vi "Image to Printer.vi"(8 "error in (no error)":errorcluster, 11 "Control Ref Queue":T1) -> (0 "error out":errorcluster)   [LabVIEW 2017, in "3D Plot.lvclass"]
uses:
  <vilib>/Math Plots/3D Math Plots/3D Plot/3D Plot/3D Plot.lvclass
  <vilib>/Math Plots/3D Math Plots/3D Plot/Action String/3DMathPlot Ctrl Act Queue.ctl
  <vilib>/Math Plots/3D Math Plots/3D Plot/Action String/3DMathPlot Ctrl Act Cluster.ctl
  <vilib>/Math Plots/3D Math Plots/3D Plot/Action String/3DMathPlot State Class.ctl
  <vilib>/Math Plots/Plot Private Lib/NI_Math Plot Private Lib.lvlib
panel:
  in  "Print Image":picture
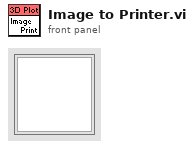
[diagram p1: front panel]
types:
  T1 = typedef "3DMathPlot Ctrl Act Queue.ctl" = refnum<queue>
  T2 = typedef "3DMathPlot Ctrl Act Cluster.ctl" = cluster{"3D Picture Control":refnum<vi>, "Render Window Refnum":refnum<vi>, "XY Graph":refnum<vi>, "Intensity Graph":refnum<vi>, "Color Legend Palette":refnum<vi>, "Projection Palette":refnum<vi>, "XControl  Ref":refnum<vi>, "Facade Ref":refnum<vi>, "Export Image Ref":refnum<vi>, "Clear Data Flag":bool, "Display State Change Class":T3}
  T3 = typedef "3DMathPlot State Class.ctl" = enum16{"Update All Objects (Undo)", "Update Light Object Only", "Update Axis Object Only", "Update Plot Object Only", "Update Cursor Object Only", "Update Axis Plot Cursor Objects", "No Update"}
  T4 = typedef "imagedata.ctl" = cluster{"image type":i32, "image depth":i32, "image":u8[], "mask":u8[], "colors":u32[], "Rectangle":cluster{"left":i16, "top":i16, "right":i16, "bottom":i16}}
  T5 = typedef "LVRectTypeDef.ctl" = cluster{"Left":i16, "Top":i16, "Right":i16, "Bottom":i16}
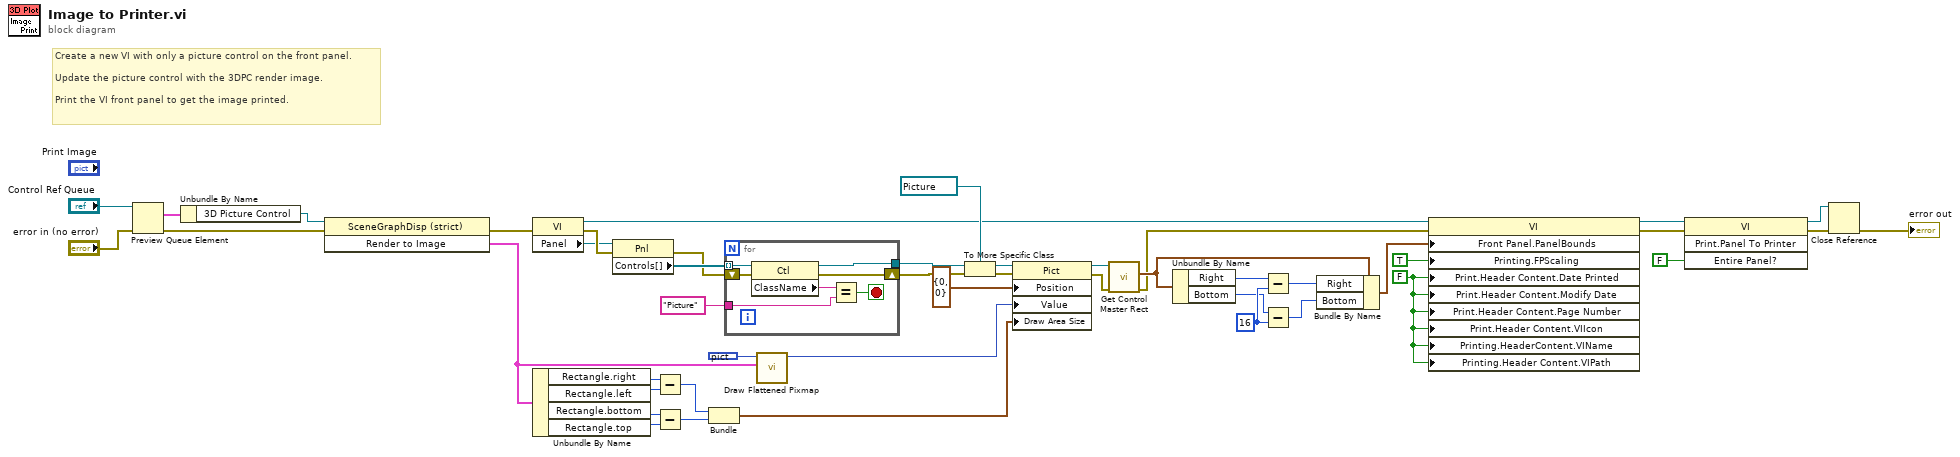
[diagram p0: block diagram]
diagram:
  w20 = i16 16
  w31 = FALSE ("Printing:Front Panel Scaling?")
  # "Create a new VI with only a picture control on the front panel.\n\nUpdate the picture control with the 3DPC render image.\n\nPrint the VI front panel to get the image printed."
  n1 = Preview Queue Element(queue="Control Ref Queue", error in (no error)="error in (no error)") -> (element=w28:T2, error out=w26:errorcluster)  [unwired: 3 out]
  n2 = Unbundle By Name(w28) -> ("3D Picture Control"=w27:refnum<vi>)
  n3 = invoke on="Invoke Node" class="SceneGraphDisp (strict)" method="Render to Image"(reference=w27, error in=w26) -> (error out=w13:errorcluster, "Get Image"=w29:T4)  [unwired: 1 in, 1 out]
  n4 = property class="VI"(error in=w13) -> (reference out=w14:refnum<vi>, error out=w16:errorcluster, "Panel"=w15:refnum<vi>)  [unwired: 1 in]
  n5 = Unbundle By Name(w29) -> ("Rectangle.right"=w38:i16, "Rectangle.left"=w40:i16, "Rectangle.bottom"=w37:i16, "Rectangle.top"=w39:i16)
  n6 = property class="Pnl"(reference=w15, error in=w16) -> (error out=w4:errorcluster, "Controls[]"=w6:refnum<vi>[])  [unwired: 1 out]
  n7 = Subtract(x=w38, y=w40) -> (x-y=w42:i16)
  n8 = Subtract(x=w37, y=w39) -> (x-y=w41:i16)
  n9 = Bundle(w42, w41) -> (w2:cluster{i16, i16})  [unwired: 1 out]
  n10 = for {
    tunnel: w6 -> [w53] mode=indexing
    tunnel: [w50] -> w5
    shift-right: [w48] -> w3
    shift-left: w4 -> [w49]
    tunnel: "Picture" -> [w47]
    stop <- w51 stop-if-true
    n11 = property class="Ctl"(reference=w53, error in=w49) -> (reference out=w50:refnum<vi>, error out=w48:errorcluster, "ClassName"=w52:string)
    n12 = Equal?(x=w52, y=w47) -> (x = y?=w51:bool)
  }
  n13 = call <vilib>:"Draw Flattened Pixmap.vi"("image data"=w29, "picture"=picture data[5B]) -> ("new picture"=w8:picture)  [unwired: 7 out]
  n14 = To More Specific Class(target class=refnum<vi> refnum ("reference"), reference=w5, error in=w3) -> (specific class reference=w24:refnum<vi>, error out=w25:errorcluster)
  n15 = property class="Pict"(reference=w24, error in=w25, "Position"=cluster{"Horizontal":i16, "Vertical":i16} {"Horizontal"=0, "Vertical"=0} ("relative position/next to refnum"), "Value"=w8, "Draw Area Size"=w2) -> (reference out=w12:refnum<vi>, error out=w11:errorcluster)
  n16 = call <vilib>:"Get Control Master Rect.vi"("error in (no error)"=w11, "reference"=w12) -> ("error out"=w7:errorcluster, "Master Bounds Rect"=w10:T5)  [unwired: 8 in]
  n17 = Unbundle By Name(w10) -> ("Right"=w21:i16, "Bottom"=w19:i16)
  n18 = Subtract(x=w21, y=w20) -> (x-y=w17:i16)
  n19 = Subtract(x=w19, y=w20) -> (x-y=w18:i16)
  n20 = Bundle By Name(cluster=w10, "Right"=w17, "Bottom"=w18) -> (w9:T5)
  n21 = property class="VI"(reference=w14, error in=w7, "Front Panel.PanelBounds"=w9, "Printing.FPScaling"=TRUE ("Printing:Front Panel Scaling?"), "Print.Header Content.Date Printed"=w31, "Print.Header Content.Modify Date"=w31, "Print.Header Content.Page Number"=w31, "Print.Header Content.VIIcon"=w31, "Printing.HeaderContent.VIName"=w31, "Printing.Header Content.VIPath"=w31) -> (reference out=w34:refnum<vi>, error out=w33:errorcluster)
  n22 = invoke class="VI" method="Print.Panel To Printer"(reference=w34, error in=w33, "Entire Panel?"=FALSE) -> (reference out=w36:refnum<vi>, error out=w35:errorcluster)  [unwired: 1 in, 2 out]
  n23 = Close Reference(reference=w36, error in (no error)=w35) -> (error out=→"error out":errorcluster)
